vi "String Less Than Ignore Case.vi"(1 "String 2":string, 2 "String":string) -> (0 "less?":bool)   [LabVIEW 2023]
doc: "Compares two strings for whether one is less than the other, ignoring case."
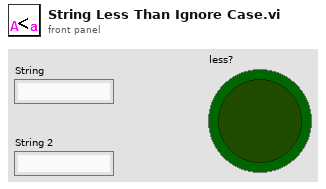
[diagram p1: front panel]
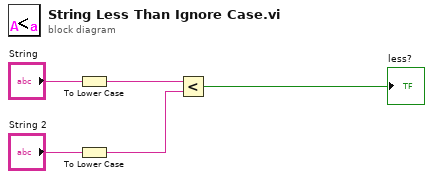
[diagram p0: block diagram]
diagram:
  n1 = To Lower Case(string="String") -> (all lower case string=w1:string)
  n2 = To Lower Case(string="String 2") -> (all lower case string=w4:string)
  n3 = Less?(x=w1, y=w4) -> (x < y?=→"less?":bool)
